vi "Revision Query.vi"(0 "VISA resource name":refnum<visa-resource-name>, 11 "error in (no error)":errorcluster) -> (4 "VISA resource name out":refnum<visa-resource-name>, 6 "Instr Serial Number":string, 8 "Instr Driver Revision":string, 10 "Instr Firmware Revision":string, 14 "Instr Model Number":string, 15 "error out":errorcluster)   [LabVIEW 2021, in "Lake Shore Cryotronics 340.lvlib"]
doc: "This VI queries the current instrument firmware revision and instrument driver revision.\nThis Instrument Driver's Revision number is \"REV 1.0, 06/1999, LV 5.0\" and is compatible with Instrument Firmware Revision: \"01.01.09\" and later.\n\nLakeShore Cryotronics Model 340 Temperature Controller\nCreated By: Rob Welsh\nRelease Date: June 1999\nOriginally Developed in LabVIEW Version: 5.0\n\nModification History: \n\nNone"
uses:
  Lake Shore Cryotronics 340.lvlib
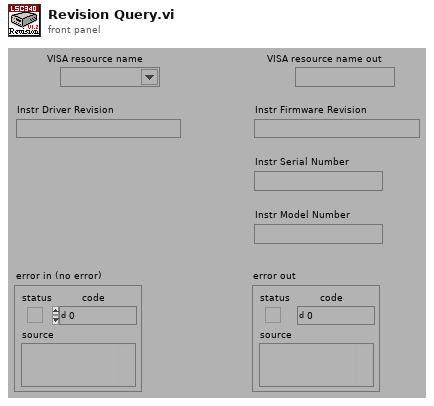
[diagram p1: front panel]
types:
  T1 = enum32{"invalid app kind", "Development System", "Run Time System", "Student Edition", "Embedded LabVIEW", "Evaluation", "Custom"}
  T2 = cluster{"Major":u16, "Minor":u16, "Fix":u16, "Build":u16}
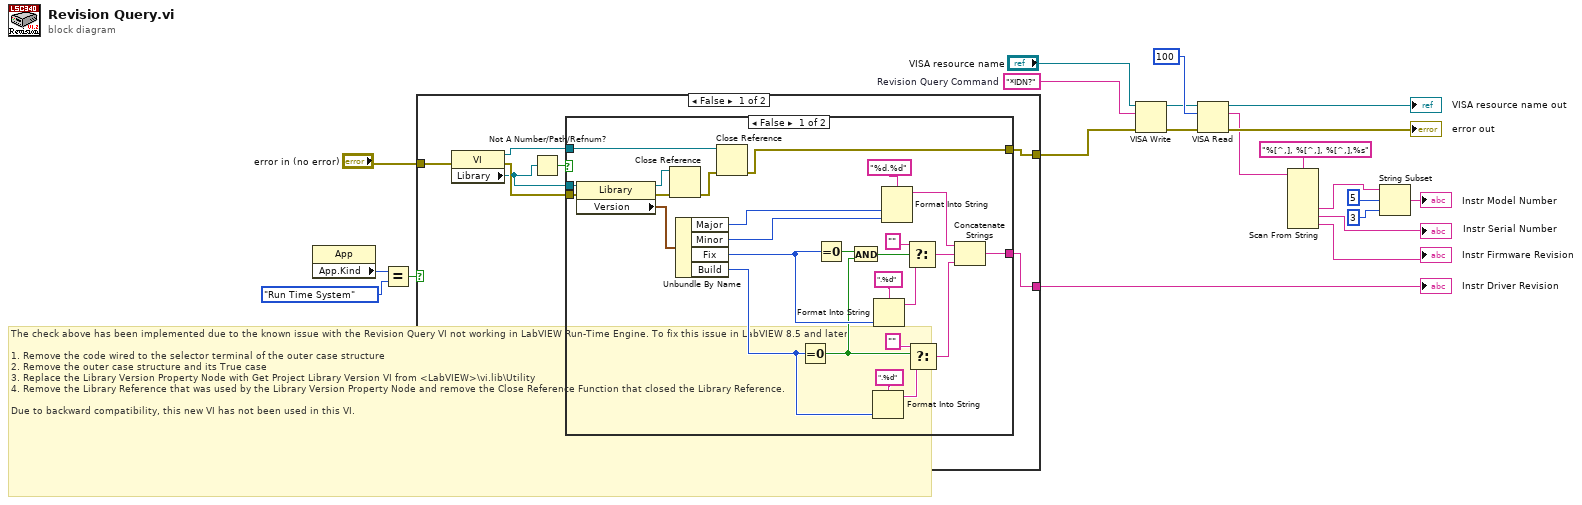
[diagram p0: block diagram]
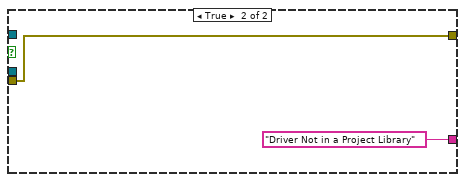
[diagram p2: hidden frame]
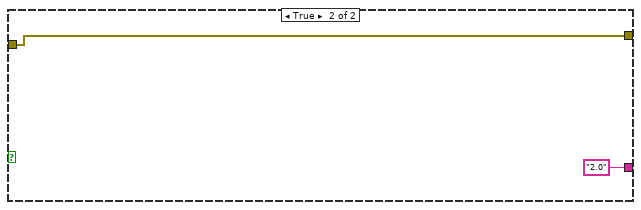
[diagram p3: hidden frame]
diagram:
  w15 = "*IDN?"  # Revision Query Command
  # "The check above has been implemented due to the known issue with the Revision Query VI not working in LabVIEW Run-Time Engine. To fix this issue in LabVIEW 8.5 and later:\n\n1. Remove the code wired to the selector terminal of the outer case structure\n2. Remove the outer case structure and its True case\n3. Replace the Library Version Property Node with Get Project Library Version VI from <LabVIEW>\\vi.lib\\Utility\n4. Remove the Library Reference that was used by the Library Version Property Node and remove the Close Reference Function that closed the Library Reference.\n\nDue to backward compatibility, this new VI has not been used in this VI."
  n1 = property class="App"() -> ("App.Kind"=w2:T1)  [unwired: 2 in, 2 out]
  n2 = Equal?(x=w2, y=T1."Run Time System") -> (x = y?=w3:bool)
  n3 = case shown="False" w3 {
    tunnel: "error in (no error)" -> [w28 w58]
    tunnel: [w23 "2.0"] -> w5
    tunnel: [w22 w58] -> w4
    frame False {
      n4 = property class="VI"(error in=w28) -> (reference out=w24:refnum<vi>, error out=w27:errorcluster, "Library"=w26:refnum<vi>)  [unwired: 1 in]
      n5 = Not A Number/Path/Refnum?(number/path/refnum=w26) -> (NaN/Path/Refnum?=w25:bool)
      n6 = case shown="False" w25 {
        tunnel: [w33 w55] -> w22
        tunnel: [w32 "Driver Not in a Project Library"] -> w23
        tunnel: w27 -> [w31 w55]
        tunnel: w26 -> [w30 _]
        tunnel: w24 -> [w29 _]
        frame False {
          n7 = property class="Library"(reference=w30, error in=w31) -> (reference out=w53:refnum<vi>, error out=w54:errorcluster, "Version"=w51:T2)
          n8 = Close Reference(reference=w53, error in (no error)=w54) -> (error out=w52:errorcluster)
          n9 = Unbundle By Name(w51) -> ("Major"=w40:u16, "Minor"=w39:u16, "Fix"=w37:u16, "Build"=w38:u16)
          n10 = Close Reference(reference=w29, error in (no error)=w52) -> (error out=w33:errorcluster)
          n11 = Equal To 0?(x=w38) -> (x = 0?=w35:bool)
          n12 = Equal To 0?(x=w37) -> (x = 0?=w36:bool)
          n13 = And(x=w36, y=w35) -> (x .and. y?=w34:bool)
          n14 = Format Into String(format string=".%d", w38) -> (resulting string=w44:string)  [unwired: 2 in, 1 out]
          n15 = Format Into String(format string=".%d", w37) -> (resulting string=w48:string)  [unwired: 2 in, 1 out]
          n16 = Format Into String(format string="%d.%d", w40, w39) -> (resulting string=w46:string)  [unwired: 2 in, 1 out]
          n17 = Select(t="", s=w34, f=w48) -> (s? t:f=w45:string)
          n18 = Select(t="", s=w35, f=w44) -> (s? t:f=w41:string)
          n19 = Concatenate Strings(w46, w45, w41) -> (w32:string)
        }
        frame True {
        }
      }
    }
    frame True {
    }
  }
  "Instr Driver Revision" <- w5
  n20 = VISA Write(VISA resource name="VISA resource name", write buffer=w15, error in (no error)=w4) -> (VISA resource name out=w17:refnum<visa-resource-name>, error out=w16:errorcluster)  [unwired: 1 out]
  n21 = VISA Read(VISA resource name=w17, byte count=u32 100 ("Num Bytes to Read"), error in (no error)=w16) -> (VISA resource name out=→"VISA resource name out":refnum<visa-resource-name>, read buffer=w10:string, error out=→"error out":errorcluster)  [unwired: 1 out]
  n22 = Scan From String(format string="%[^,], %[^,], %[^,],%s", input string=w10) -> (output 2=w13:string, output 3=→"Instr Serial Number":string, output 4=→"Instr Firmware Revision":string)  [unwired: 7 in, 3 out]
  n23 = String Subset(string=w13, offset (0)=5, length (rest)=3) -> (substring=→"Instr Model Number":string)
